vi "Pair with Nearest.vi"(8 "error in (no error)":errorcluster, 11 "State in":T1={"Raw File Data"="", "Deduplicated String Array"=[], "1-Entries"=[], "2-Entries"=[], "3-Entries"=[], "Bounds"={"M-Min"=0, "M-Max"=1023, "S-Min"=0, "S-Max"=1023}, "Matched ADC Values - Nearest"=[], "Match Entry Indices - Nearest"=[], "Filtered 1-Entries"=[], "Filtered 2-Entries"=[], "Filtered 3-Entries"=[], "Total Duration"=0.0, "Matched ADC Values - Largest"=[], "Match Entry Indices - Largest"=[], "Unmatched 1-Entries - Nearest"=[], "Unmatched 1-Entries - Largest"=[]}) -> (0 "error out":errorcluster, 3 "State out":T1={"Raw File Data"="", "Deduplicated String Array"=[], "1-Entries"=[], "2-Entries"=[], "3-Entries"=[], "Bounds"={"M-Min"=0, "M-Max"=1023, "S-Min"=0, "S-Max"=1023}, "Matched ADC Values - Nearest"=[], "Match Entry Indices - Nearest"=[], "Filtered 1-Entries"=[], "Filtered 2-Entries"=[], "Filtered 3-Entries"=[], "Total Duration"=0.0, "Matched ADC Values - Largest"=[], "Match Entry Indices - Largest"=[], "Unmatched 1-Entries - Nearest"=[], "Unmatched 1-Entries - Largest"=[]})   [LabVIEW 2019, in "Muon Data Post-Processing.lvlib"]
uses:
  Muon Data Post-Processing.lvlib
  State Data.ctl
  File Entry.ctl
  ADC Bounds.ctl
panel:
  out "Dup Match Count":i16
  out "Array":bool[](array[boolean])
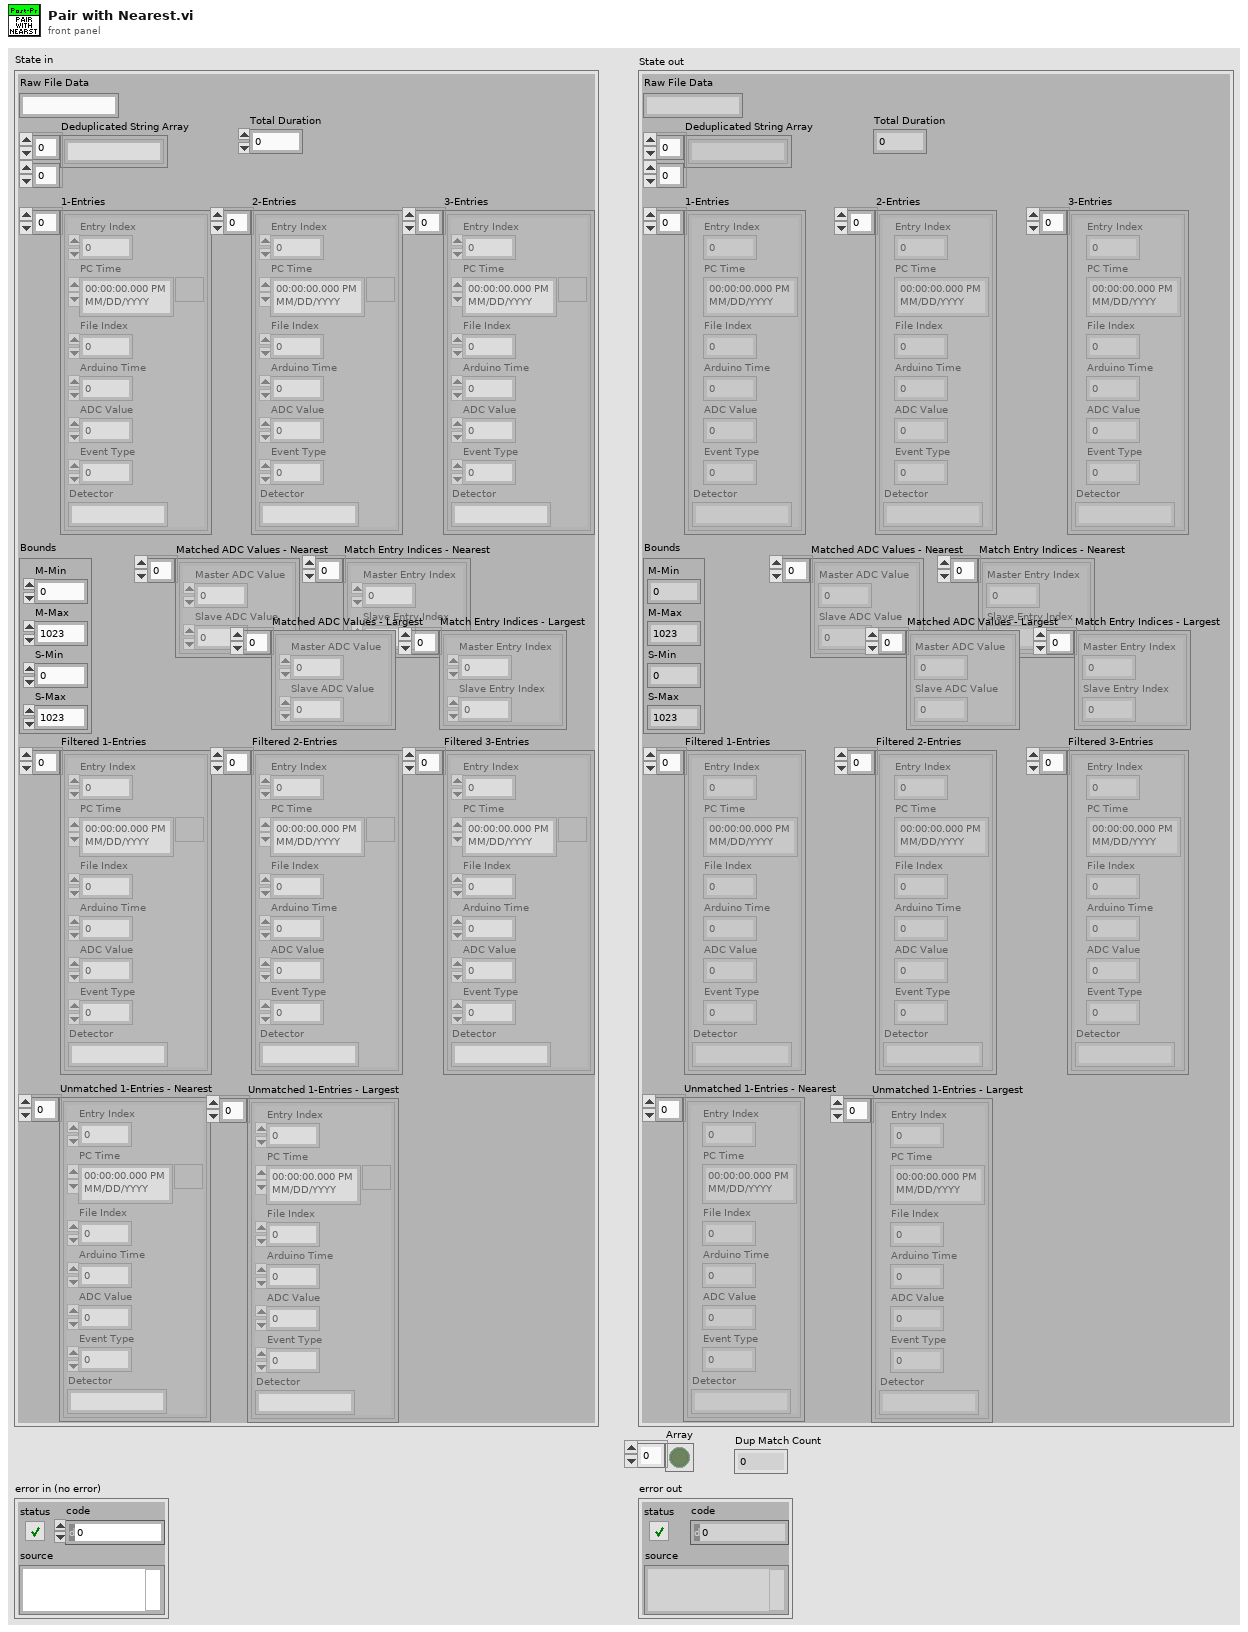
[diagram p1: front panel]
types:
  T1 = typedef "Muon Data Post-Processing.lvlib/State Data.ctl" = cluster{"Raw File Data":string, "Deduplicated String Array":string[][], "1-Entries":T2[], "2-Entries":T2[], "3-Entries":T2[], "Bounds":T3, "Matched ADC Values - Nearest":cluster{"Master ADC Value":i32, "Slave ADC Value":i32}[], "Match Entry Indices - Nearest":cluster{"Master Entry Index":i32, "Slave Entry Index":i32}[], "Filtered 1-Entries":T2[], "Filtered 2-Entries":T2[], "Filtered 3-Entries":T2[], "Total Duration":dbl, "Matched ADC Values - Largest":cluster{"Master ADC Value":i32, "Slave ADC Value":i32}[], "Match Entry Indices - Largest":cluster{"Master Entry Index":i32, "Slave Entry Index":i32}[], "Unmatched 1-Entries - Nearest":T2[], "Unmatched 1-Entries - Largest":T2[]}
  T2 = typedef "Muon Data Post-Processing.lvlib/File Entry.ctl" = cluster{"Entry Index":i32, "PC Time":timestamp, "File Index":i32, "Arduino Time":i32, "ADC Value":i32, "Event Type":i32, "Detector":string}
  T3 = typedef "Muon Data Post-Processing.lvlib/ADC Bounds.ctl" = cluster{"M-Min":u16, "M-Max":u16, "S-Min":u16, "S-Max":u16}
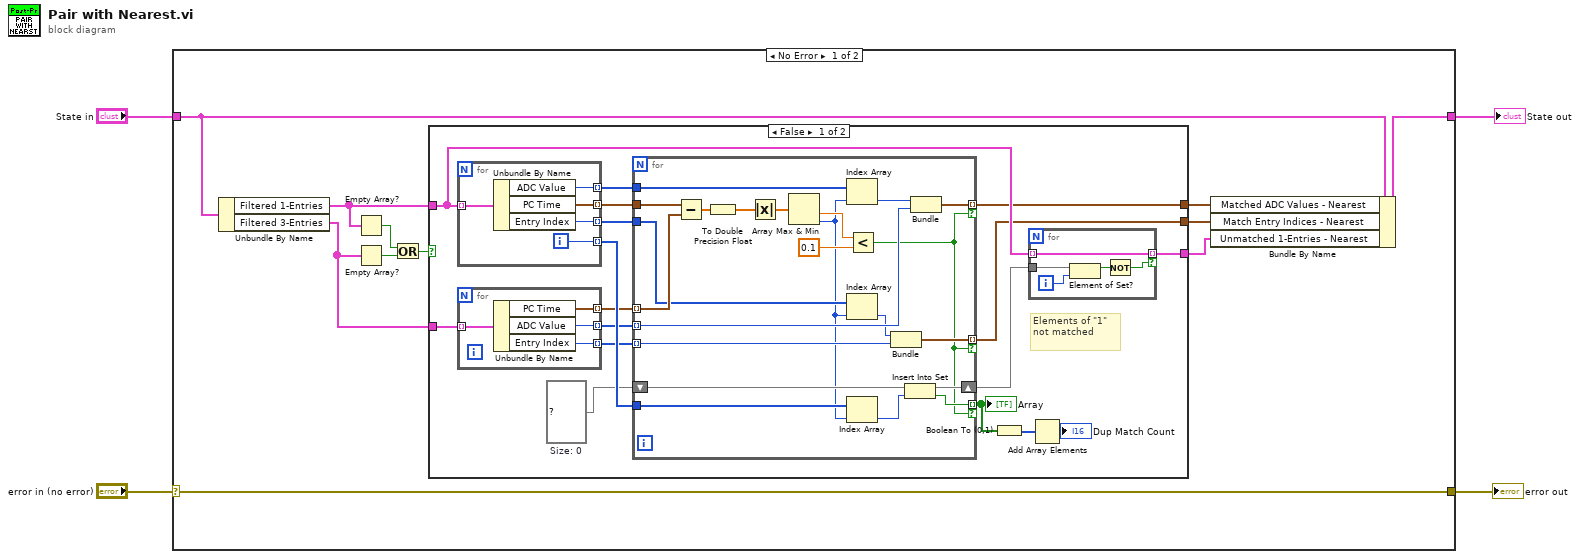
[diagram p0: block diagram]
diagram:
  n1 = case shown="No Error" "error in (no error)" {
    selector: "error in (no error)" -> [w14 w70]
    tunnel: [w13 w71] -> w3
    tunnel: "State in" -> [w15 w71]
    tunnel: [w14 w70] -> w1
    frame No Error {
      n2 = Unbundle By Name(w15) -> ("Filtered 1-Entries"=w10:T2[], "Filtered 3-Entries"=w9:T2[])
      n3 = Empty Array?(array=w10) -> (empty?=w8:bool)
      n4 = Empty Array?(array=w9) -> (empty?=w7:bool)
      n5 = Or(x=w8, y=w7) -> (x .or. y?=w6:bool)
      n6 = case shown="False" w6 {
        tunnel: [w24 _] -> w12
        tunnel: [w23 _] -> w11
        tunnel: w10 -> [w32 w69]
        tunnel: w9 -> [w22 _]
        tunnel: [w19 w69] -> w5
        frame False {
          w21 = set{i32} {}  # Size: 0
          # "Elements of \"1\" not matched"
          n7 = for {
            tunnel: w32 -> [w68] mode=indexing
            tunnel: [w67] -> w30 mode=indexing
            tunnel: [w66] -> w29 mode=indexing
            tunnel: [w65] -> w25 mode=indexing
            tunnel: [w64] -> w31 mode=indexing
            i -> [w64]
            n8 = Unbundle By Name(w68) -> ("ADC Value"=w65:i32, "PC Time"=w67:timestamp, "Entry Index"=w66:i32)
          }
          n9 = for {
            tunnel: w22 -> [w63] mode=indexing
            tunnel: [w62] -> w28 mode=indexing
            tunnel: [w61] -> w27 mode=indexing
            tunnel: [w60] -> w26 mode=indexing
            n10 = Unbundle By Name(w63) -> ("PC Time"=w62:timestamp, "ADC Value"=w60:i32, "Entry Index"=w61:i32)
          }
          n11 = for {
            tunnel: w30 -> [w53]
            tunnel: w29 -> [w51]
            tunnel: w28 -> [w52] mode=indexing
            tunnel: w27 -> [w50] mode=indexing
            tunnel: [w49] -> w23 mode=indexing if=w38
            tunnel: w26 -> [w46] mode=indexing
            tunnel: w25 -> [w48]
            tunnel: [w45] -> w24 mode=indexing if=w38
            tunnel: w31 -> [w59]
            shift-right: [w42] -> w20
            shift-left: w21 -> [w43]
            tunnel: [w39] -> w16 mode=indexing if=w38
            n12 = Subtract(x=w53, y=w52) -> (x-y=w58:dbl[])
            n13 = To Double Precision Float(number=w58) -> (double precision float=w57:dbl[])
            n14 = Absolute Value(x=w57) -> (abs(x)=w55:dbl[])
            n15 = Array Max & Min(array=w55) -> (min value=w54:dbl, min index (indices)=w41:i32)  [unwired: 2 out]
            n16 = Index Array(array=w48, index=w41) -> (element=w47:i32)
            n17 = Index Array(array=w51, index=w41) -> (element=w44:i32)
            n18 = Index Array(array=w59, index=w41) -> (element=w40:i32)
            n19 = Less?(x=w54, y=0.1) -> (x < y?=w38:bool)
            n20 = Bundle("Entry Index"=w44, "Entry Index"=w50) -> (w49:cluster{"Entry Index":i32, "Entry Index":i32})  [unwired: 1 in]
            n21 = Insert Into Set(10:w40, 11:w43) -> (2:w39:bool, 3:w42:set{i32})
            n22 = Bundle("ADC Value"=w47, "ADC Value"=w46) -> (w45:cluster{"ADC Value":i32, "ADC Value":i32})  [unwired: 1 in]
          }
          "Array" <- w16
          n23 = Boolean To (0,1)(Boolean=w16) -> (0, 1=w18:i16[])
          n24 = for {
            tunnel: w32 -> [w35] mode=indexing
            tunnel: w20 -> [w37]
            tunnel: [w35] -> w19 mode=indexing if=w33
            i -> [w36]
            n25 = Element of Set?(10:w36, 11:w37) -> (3:w34:bool)
            n26 = Not(x=w34) -> (.not. x?=w33:bool)
          }
          n27 = Add Array Elements(numeric array=w18) -> (sum=→"Dup Match Count":i16)
        }
        frame True {
        }
      }
      n28 = Bundle By Name(cluster=w15, "Matched ADC Values - Nearest"=w12, "Match Entry Indices - Nearest"=w11, "Unmatched 1-Entries - Nearest"=w5) -> (w13:T1)
    }
    frame Error {
    }
  }
  "State out" <- w3
  "error out" <- w1
